vi "ReadIOMerge.vi"   [LabVIEW 2020]
doc: "Reads the I/O data from the I/O items. This function waits for new I/O data to become available through the Generate I/O Sample Pulse Method function."
uses:
  <vilib>/eio/EIOGrowableMethodNode/genericMethod/EIOGrowableMethodNode.xnode
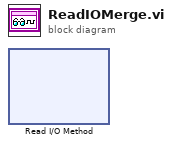
[diagram p0: block diagram]
diagram:
  n1 = xnode "Read I/O Method"() -> ()  [unwired: 2 in, 3 out]
